vi "kalman pv cycle fixed gain.vi"(8 "v gain":fxp<+,16,0>=0.136993408203125 format="%.16g", 9 "x gain":fxp<+,16,0>=0.4766998291015625 format="%.16g", 10 "position measurement":i16, 11 "Kalman PV state":T1) -> (3 "kalman pv state out":T1)   [LabVIEW 2010]
uses:
  kalman pv state.ctl
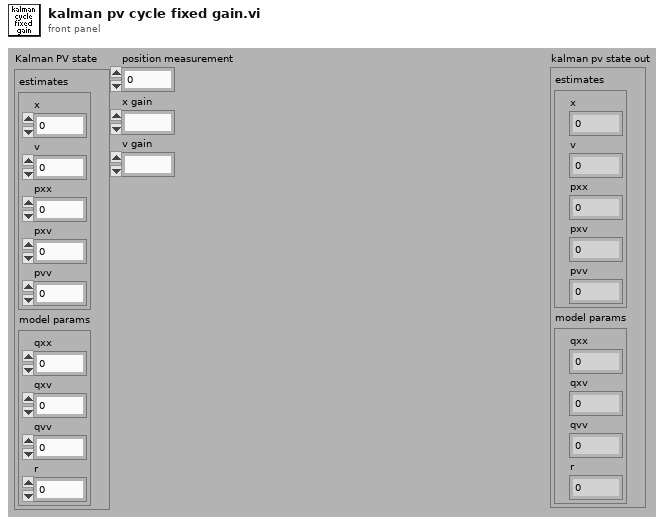
[diagram p1: front panel]
types:
  T1 = typedef "kalman pv state.ctl" = cluster{"estimates":cluster{"x":fxp<+/-,18,16>, "v":fxp<+/-,18,16>, "pxx":u16, "pxv":u16, "pvv":u16}, "model params":cluster{"qxx":u16, "qxv":u16, "qvv":u16, "r":u16}}
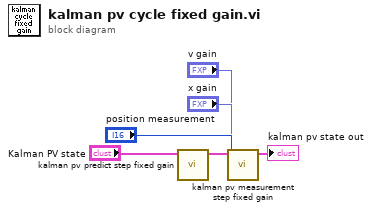
[diagram p0: block diagram]
diagram:
  n1 = call "kalman pv predict step fixed gain.vi"("Kalman PV state"="Kalman PV state") -> ("Kalman PV state out"=w6:T1)  [unwired: 10 in]
  n2 = call "kalman pv measurement step fixed gain.vi"("v gain"="v gain", "x gain"="x gain", "position measurement"="position measurement", "Kalman PV state"=w6) -> ("kalman pv state out"=→"kalman pv state out":T1)  [unwired: 7 in]
